vi "Instrument Set Timeout.vi"(0 "Reference In":refnum<visa-resource-name>, 5 "Timeout Value":u32=2000, 11 "error in (no error)":errorcluster) -> (4 "reference out":refnum<visa-resource-name>, 15 "error out":errorcluster)   [LabVIEW 2018]
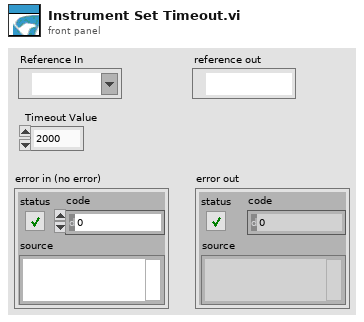
[diagram p1: front panel]
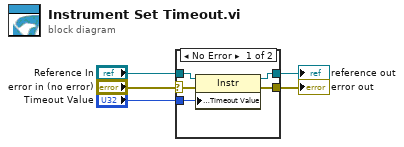
[diagram p0: block diagram]
diagram:
  n1 = case shown="No Error" "error in (no error)" {
    selector: "error in (no error)" -> [w10 w12]
    tunnel: [w7 w12] -> w4
    tunnel: "Timeout Value" -> [w9 _]
    tunnel: [w8 w11] -> w2
    tunnel: "Reference In" -> [w6 w11]
    frame No Error {
      n2 = property class="Instr"(reference=w6, error in=w10, "General Settings:Timeout Value"=w9) -> (reference out=w8:refnum<visa-resource-name>, error out=w7:errorcluster)
    }
    frame Error {
    }
  }
  "error out" <- w4
  "reference out" <- w2
